vi "Stop Pat GV.vi"() -> ()   [LabVIEW 2026]
panel:
  in  "Stop Pat":bool
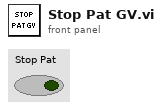
[diagram p1: front panel]
diagram:
